vi "Untitled 6.vi"() -> ()   [LabVIEW 2023]
uses:
  Controls/Queue_Operation_Select.ctl
  Controls/State_and_Data.ctl
  Controls/Notifier_Operation_Select.ctl
panel:
  in  "Error_In":errorcluster
  in  "File_hierarchy":string(tree)
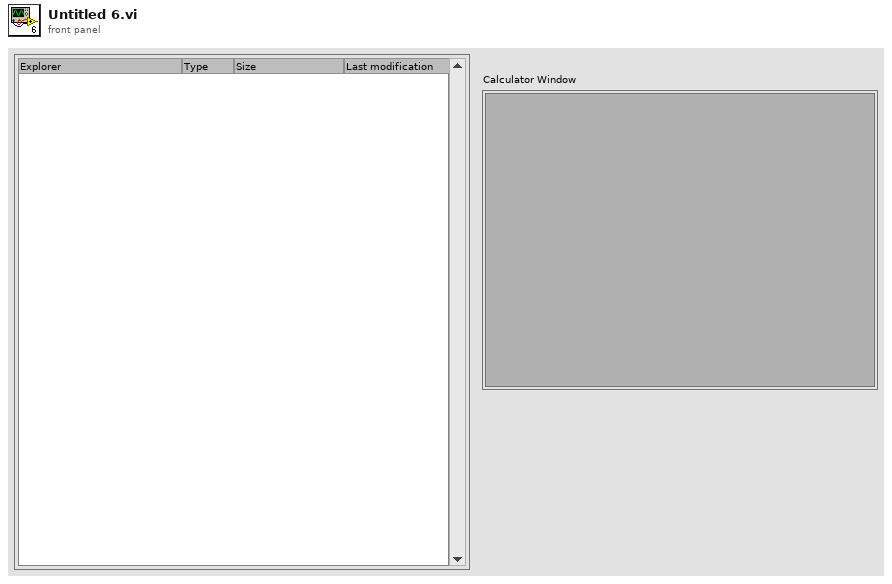
[diagram p1: front panel]
types:
  T1 = typedef "Notifier_Operation_Select.ctl" = enum16{"Obtain_Notifier", "Send_Notification", "Get_Notification_Status", "Release_Notifier"}
  T2 = typedef "State_and_Data.ctl" = cluster{"State":string, "Data":variant}
  T3 = cluster{"File_hierarchy_Reference":refnum<vi>, "Tag":string, "State_and_Data":T2}
  T4 = typedef "Queue_Operation_Select.ctl" = enum16{"Obtain_Queue", "Enqueue", "Enqueue_First", "Enqueue_N", "Lossy_Enqueue", "Preview", "Queue_Status", "Dequeue", "Flush", "Release_Queue"}
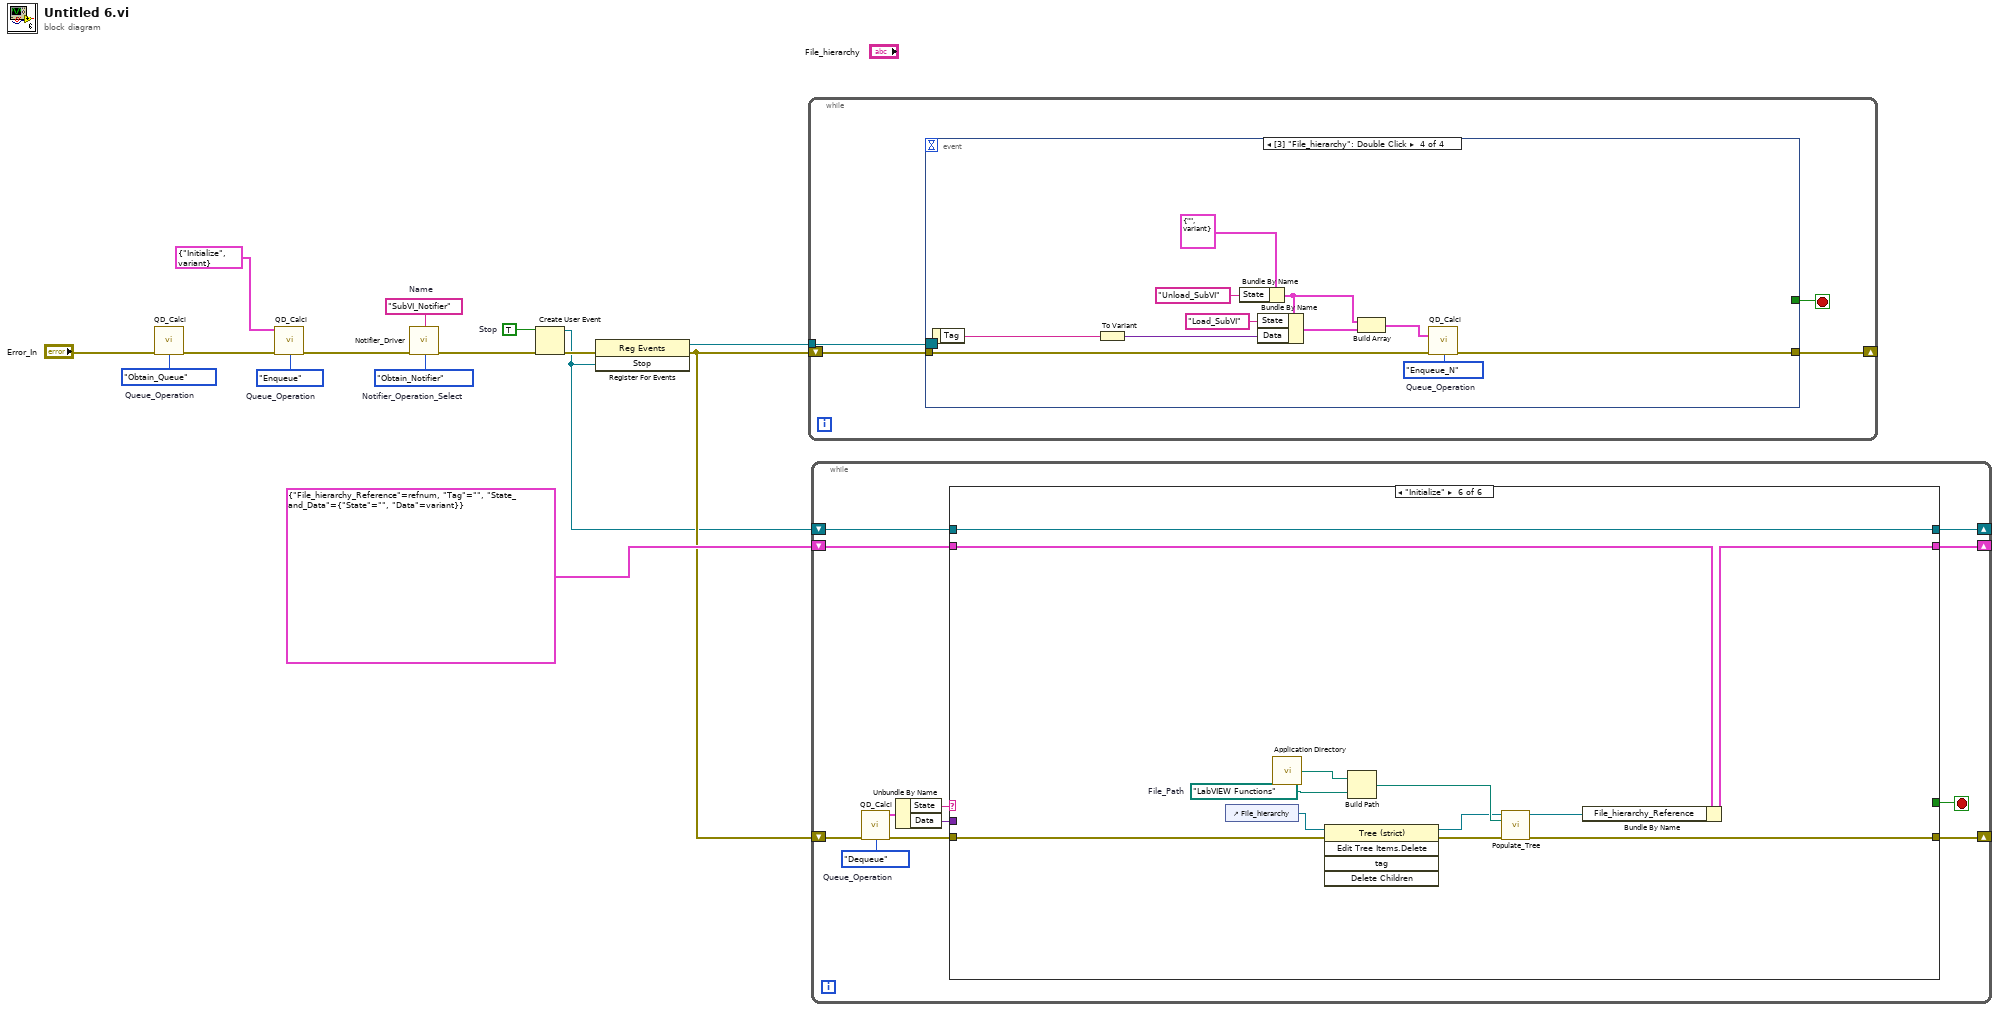
[diagram p0: block diagram]
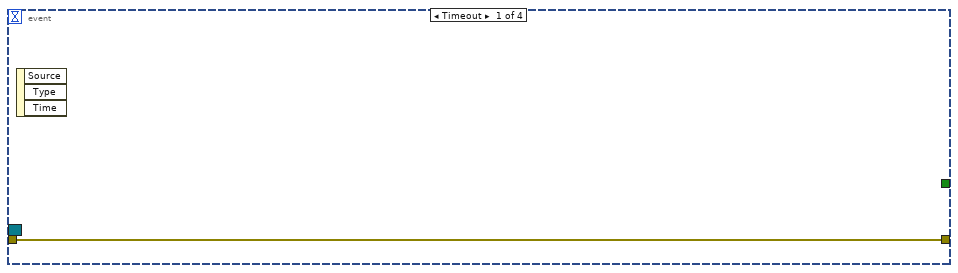
[diagram p2: hidden frame]
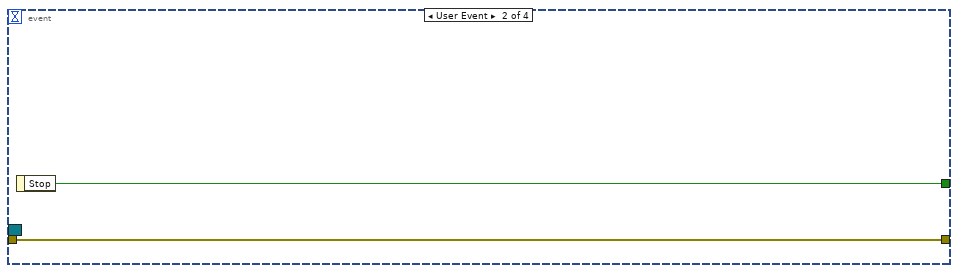
[diagram p3: hidden frame]
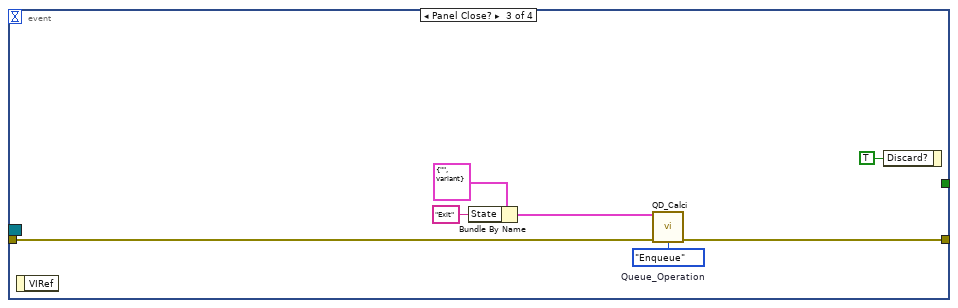
[diagram p4: hidden frame]
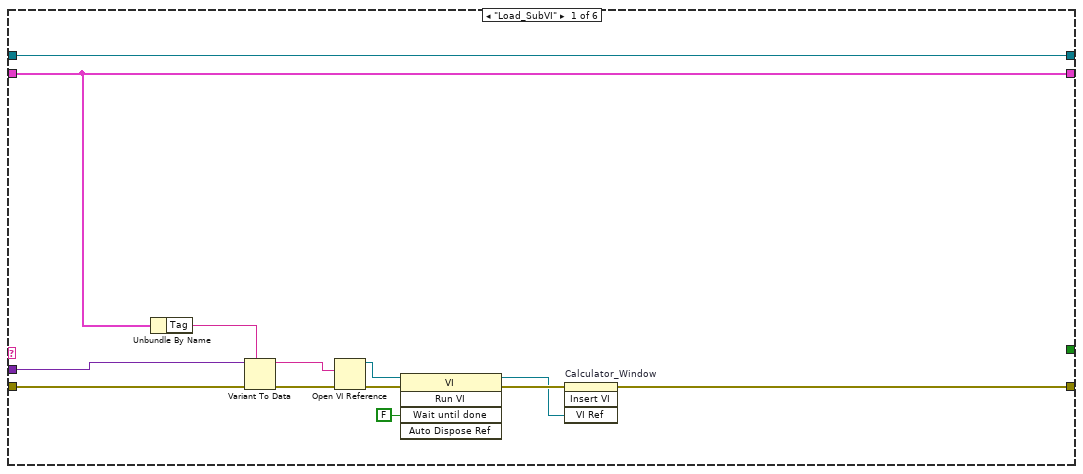
[diagram p5: hidden frame]
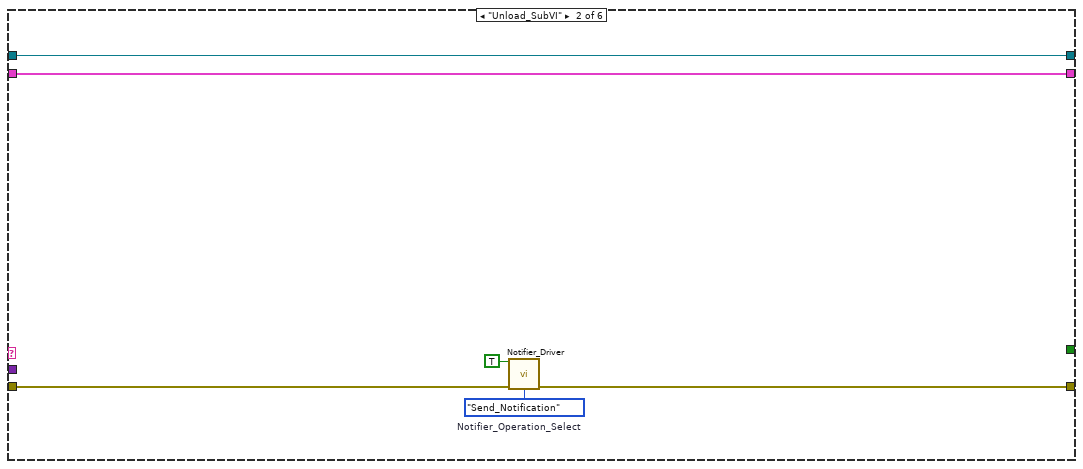
[diagram p6: hidden frame]
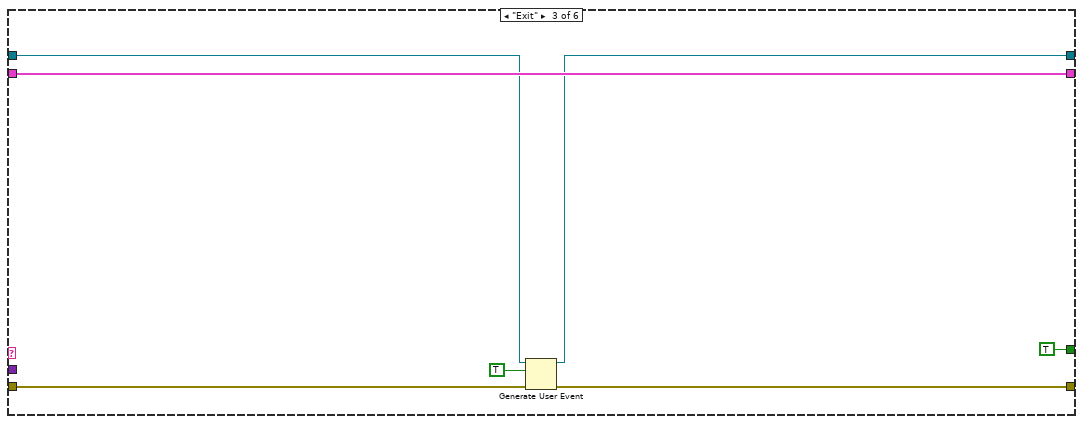
[diagram p7: hidden frame]
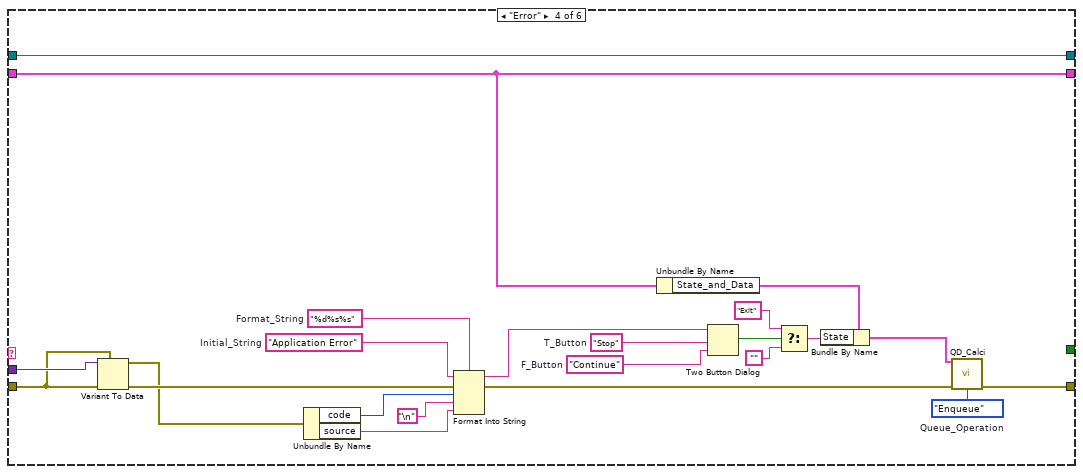
[diagram p8: hidden frame]
diagram:
  w4 = TRUE  # Stop
  w6 = "SubVI_Notifier"  # Name
  w7 = Notifier_Operation_Select."Obtain_Notifier"  # Notifier_Operation_Select
  w12 = Queue_Operation_Select."Enqueue"  # Queue_Operation
  w13 = Queue_Operation_Select."Obtain_Queue"  # Queue_Operation
  n1 = call "QD_Calci.vi"("Error_In"="Error_In", "Queue_Operation"=w13) -> ("Error_Out"=w14:errorcluster)  [unwired: 11 in, 2 out]
  n2 = call "QD_Calci.vi"("State_and_Data_In"=T2 {"State"="Initialize", "Data"=variant} ("State_and_Data"), "Error_In"=w14, "Queue_Operation"=w12) -> ("Error_Out"=w10:errorcluster)  [unwired: 10 in, 2 out]
  n3 = call "Notifier_Driver.vi"("Name"=w6, "Error_In"=w10, "Notifier_Operation_Select"=w7) -> ("Error_Out"=w8:errorcluster)  [unwired: 11 in, 1 out]
  n4 = Create User Event(user event datatype=w4, error in=w8) -> (user event=w1:refnum<user-event>, error out=w5:errorcluster)
  n5 = register-events(error in=w5, w1) -> (reference out=w2:refnum<event-registration>, error out=w3:errorcluster)  [unwired: 1 in]
  n6 = while {
    tunnel: w2 -> [w18]
    shift-right: [w16] -> _
    shift-left: w3 -> [w19]
    stop <- w17 stop-if-true
    n7 = event shown="[3] \"File_hierarchy\": Double Click" {
      selector: w18 -> [_ _ _ _]
      dyn-events: _ -> [_ _ _ _]
      timeout: _ -> [_ _ _ _]
      tunnel: w19 -> [w20 w22 w26 w40]
      tunnel: [w20 w22 w25 w39] -> w16
      tunnel: [_ w21 _ _] -> w17
      event Timeout {
        n8 = event-data() -> ()  [unwired: 1 in, 3 out]
      }
      event User Event {
        n9 = event-data() -> ("Stop"=w21:bool)  [unwired: 1 in]
      }
      event Panel Close? {
        w27 = Queue_Operation_Select."Enqueue"  # Queue_Operation
        n10 = event-data() -> ()  [unwired: 1 in, 1 out]
        n11 = Bundle By Name(cluster=T2 {"State"="", "Data"=variant} ("State_and_Data"), "State"="Exit") -> (w24:T2)
        n12 = call "QD_Calci.vi"("State_and_Data_In"=w24, "Error_In"=w26, "Queue_Operation"=w27) -> ("Error_Out"=w25:errorcluster)  [unwired: 10 in, 2 out]
        n13 = event-data("Discard?"=TRUE) -> ()  [unwired: 1 in, 1 out]
      }
      event "File_hierarchy": Double Click {
        w35 = Queue_Operation_Select."Enqueue_N"  # Queue_Operation
        n14 = event-data() -> ("Tag"=w37:string)  [unwired: 1 in]
        n15 = To Variant(anything=w37) -> (Variant=w36:variant)
        n16 = Bundle By Name(cluster=T2 {"State"="", "Data"=variant} ("State_and_Data"), "State"="Unload_SubVI") -> (w31:T2)
        n17 = Bundle By Name(cluster=w31, "State"="Load_SubVI", "Data"=w36) -> (w32:T2)
        n18 = Build Array(w31, w32) -> (w30:T2[])
        n19 = call "QD_Calci.vi"("State_and_Data_N_In"=w30, "Error_In"=w40, "Queue_Operation"=w35) -> ("Error_Out"=w39:errorcluster)  [unwired: 10 in, 2 out]
      }
    }
  }
  n20 = while {
    shift-right: [w44] -> _
    shift-left: w1 -> [w45]
    shift-right: [w43] -> _
    shift-left: T3 {"File_hierarchy_Reference"=refnum, "Tag"="", "State_and_Data"={"State"="", "Data"=variant}} -> [w46]
    shift-right: [w42] -> _
    shift-left: w3 -> [w52]
    stop <- w41 stop-if-true
    w50 = Queue_Operation_Select."Dequeue"  # Queue_Operation
    n21 = call "QD_Calci.vi"("Error_In"=w52, "Queue_Operation"=w50) -> ("State_and_Data_Out"=w49:T2, "Error_Out"=w51:errorcluster)  [unwired: 11 in, 1 out]
    n22 = Unbundle By Name(w49) -> ("State"=w48:string, "Data"=w47:variant)
    n23 = case shown="\"Initialize\"" w48 {
      tunnel: [w62 w69 w76 w82 w104 w116] -> w42
      tunnel: w51 -> [w65 w71 w78 w99 w104 w115]
      tunnel: w47 -> [w64 _ _ w100 _ _]
      tunnel: w46 -> [w63 w70 w77 w84 w103 w108]
      tunnel: [w63 w70 w77 w84 w103 w107] -> w43
      tunnel: w45 -> [w53 w66 w75 w101 w102 w105]
      tunnel: [w53 w66 w73 w101 w102 w105] -> w44
      tunnel: [_ _ TRUE _ _ _] -> w41
      frame "Load_SubVI" {
        n24 = Unbundle By Name(w63) -> ("Tag"=w54:string)
        n25 = Variant To Data(error in=w65, type=w54, Variant=w64) -> (data=w55:string, error out=w56:errorcluster)
        n26 = Open VI Reference(vi path=w55, error in (no error)=w56) -> (vi reference=w59:refnum<vi>, error out=w61:errorcluster)  [unwired: 4 in]
        n27 = invoke class="VI" method="Run VI"(reference=w59, error in=w61, "Wait until done"=FALSE ("Wait Until Done")) -> (reference out=w58:refnum<vi>, error out=w60:errorcluster)  [unwired: 2 in, 3 out]
        n28 = invoke on="Calculator_Window" class="SubPnl" method="Insert VI"(error in=w60, "VI Ref"=w58) -> (error out=w62:errorcluster)  [unwired: 2 in, 3 out]
      }
      frame "Unload_SubVI" {
        w68 = Notifier_Operation_Select."Send_Notification"  # Notifier_Operation_Select
        n29 = call "Notifier_Driver.vi"("Notification"=TRUE, "Error_In"=w71, "Notifier_Operation_Select"=w68) -> ("Error_Out"=w69:errorcluster)  [unwired: 11 in, 1 out]
      }
      frame "Exit" {
        n30 = Generate User Event(user event=w75, event data cluster=TRUE ("event data"), error in=w78) -> (user event out=w73:refnum<user-event>, error out=w76:errorcluster)  [unwired: 1 in]
      }
      frame "Error" {
        w81 = Queue_Operation_Select."Enqueue"  # Queue_Operation
        w94 = "%d%s%s"  # Format_String
        w95 = "Application Error"  # Initial_String
        w96 = "Stop"  # T_Button
        w97 = "Continue"  # F_Button
        n31 = Variant To Data(error in=w99, type=w99, Variant=w100) -> (data=w80:errorcluster, error out=w86:errorcluster)
        n32 = Unbundle By Name(w80) -> ("code"=w92:i32, "source"=w91:string)
        n33 = Format Into String(format string=w94, initial string=w95, error in=w86, w92, "\n", w91) -> (resulting string=w98:string, error out=w85:errorcluster)
        n34 = Unbundle By Name(w84) -> ("State_and_Data"=w83:T2)
        n35 = Two Button Dialog(message=w98, 1:w97, 2:w96) -> (T button?=w89:bool)
        n36 = Select(t="Exit" ("State"), s=w89, f="") -> (s? t:f=w87:string)
        n37 = Bundle By Name(cluster=w83, "State"=w87) -> (w79:T2)
        n38 = call "QD_Calci.vi"("State_and_Data_In"=w79, "Error_In"=w85, "Queue_Operation"=w81) -> ("Error_Out"=w82:errorcluster)  [unwired: 10 in, 2 out]
      }
      frame Default {
      }
      frame "Initialize" {
        w112 = path "LabVIEW Functions"  # File_Path
        n39 = control-ref of="File_hierarchy"() -> (w110:refnum<vi>)
        n40 = call <vilib>:"Application Directory.vi"() -> ("Application Directory"=w113:path)
        n41 = invoke class="Tree (strict)" method="Edit Tree Items.Delete"(reference=w110, error in=w115) -> (reference out=w109:refnum<vi>, error out=w111:errorcluster)  [unwired: 3 in, 3 out]
        n42 = Build Path(base path=w113, name or relative path=w112) -> (appended path=w114:path)
        n43 = call "Populate_Tree.vi"("Reference_In"=w109, "File_Path"=w114, "Error_In"=w111) -> ("Reference_Out"=w106:refnum<vi>, "Error_Out"=w116:errorcluster)  [unwired: 11 in]
        n44 = Bundle By Name(cluster=w108, "File_hierarchy_Reference"=w106) -> (w107:T3)
      }
    }
  }
